vi "sm u32 write and increment.vi"(8 "error in (no error)":errorcluster, 9 "Increment value":u64=4, 10 "value in":u32, 11 "pointer in":u64) -> (0 "error out":errorcluster, 3 "Shared Memory PTR out":u64)   [LabVIEW 2018, in "linuxSharedMemory.lvlib"]
uses:
  linuxSharedMemory.lvlib
  <vilib>/NI/NI Linux RT IPC/Shared Memory/Pointer Operations/Write Scalar U32.vi
  <vilib>/NI/NI Linux RT IPC/Shared Memory/Linux RT IPC.Shared Memory.lvlib
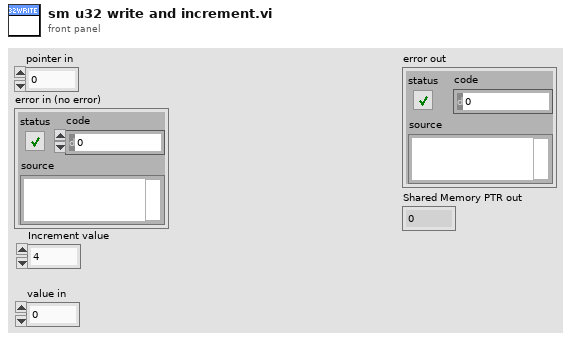
[diagram p1: front panel]
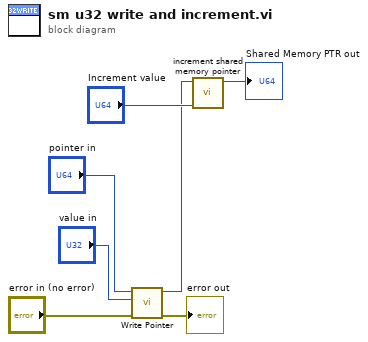
[diagram p0: block diagram]
diagram:
  n1 = call-poly <vilib>:"Write Pointer.vi"("error in (no error)"="error in (no error)", "value"="value in", "pointer in"="pointer in") -> ("error out"=→"error out":errorcluster, "pointer out"=w3:u64)  [unwired: 6 in, 1 out]
  n2 = call "increment shared memory pointer.vi"("Increment value"="Increment value", "Shared Memory PTR in"=w3) -> ("Shared Memory PTR out"=→"Shared Memory PTR out":u64)  [unwired: 9 in]
